vi "SP Read Single.vi"(8 "error in":errorcluster, 9 "Channel Index":i32=1, 11 "Current Setpoint in":refnum<class "Current Setpoint.lvclass">) -> (0 "error out":errorcluster, 1 "Changed or First Call?":bool, 2 "Current SP":dbl, 3 "Current Setpoint out":refnum<class "Current Setpoint.lvclass">)   [LabVIEW 2023, in "Current Setpoint.lvclass"]
uses:
  Current Setpoint.lvclass
  Parents/Setpoint/Setpoint.lvclass
  Current Setpoint.lvclass/Current Setpoint.ctl
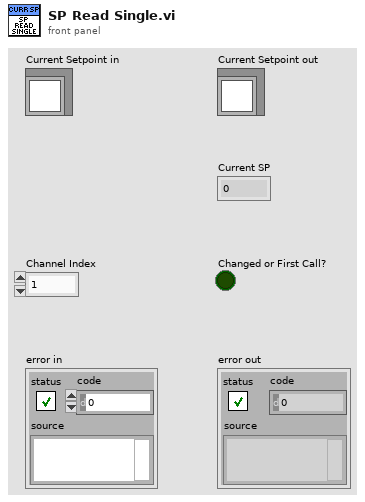
[diagram p1: front panel]
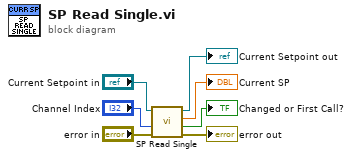
[diagram p0: block diagram]
diagram:
  n1 = call-parent "SP Read Single.vi"("error in"="error in", "Channel Index"="Channel Index", "Setpoint in"="Current Setpoint in") -> ("error out"=→"error out":errorcluster, "Changed or First Call?"=→"Changed or First Call?":bool, "Current SP"=→"Current SP":dbl, "Setpoint out"=→"Current Setpoint out":refnum<class "Current Setpoint.lvclass">)  [unwired: 5 in]
